vi "Parse Open Delimiter.vi"(8 "Error In":errorcluster, 11 "Parser In":refnum<class "Parser.lvclass">) -> (0 "Error Out":errorcluster, 3 "Parser Out":refnum<class "Parser.lvclass">)   [LabVIEW 2018, in "Toolkit.lvlib" / "Parser.lvclass"]
uses:
  Parser.lvclass
  Parser.lvclass/Parser.ctl
  API/Controls/States.ctl
  Tokens/Text/Text.lvclass
  D:/Users/cfield/Code/Field R&D Services/Mustache/trunk/src/Mustache/Public/Tokens/Public/Abstract/Abstract.lvclass
  Tokens/Text/API/New.vi
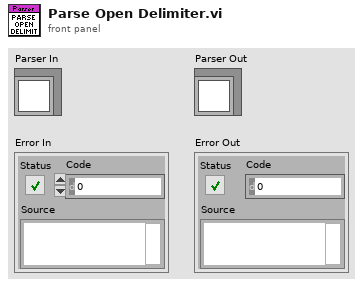
[diagram p1: front panel]
types:
  T1 = typedef "Toolkit.lvlib/Parser.lvclass/States.ctl" = enum16{"Text", "Open Delimiter", "Tag Type", "Tag Key", "Close Delimiter"}
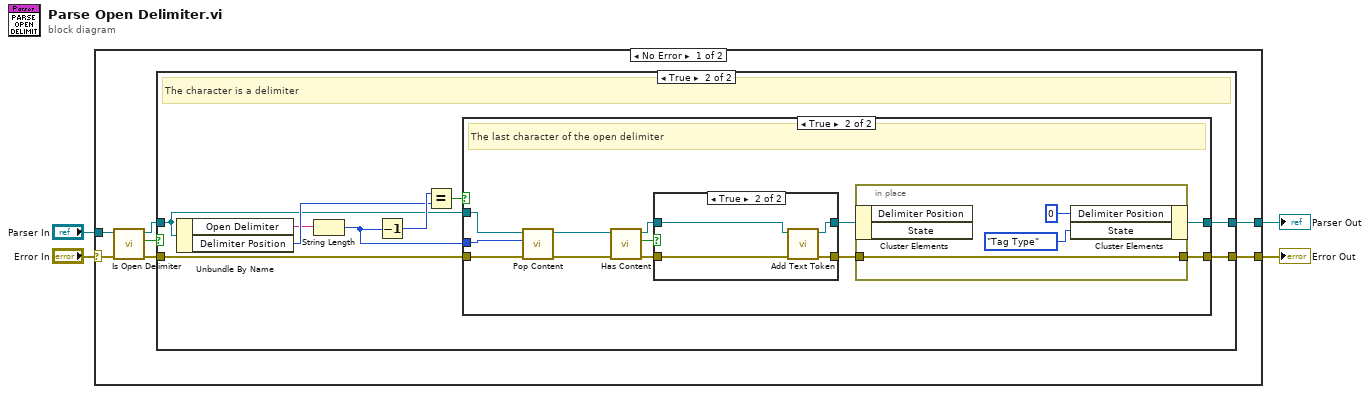
[diagram p0: block diagram]
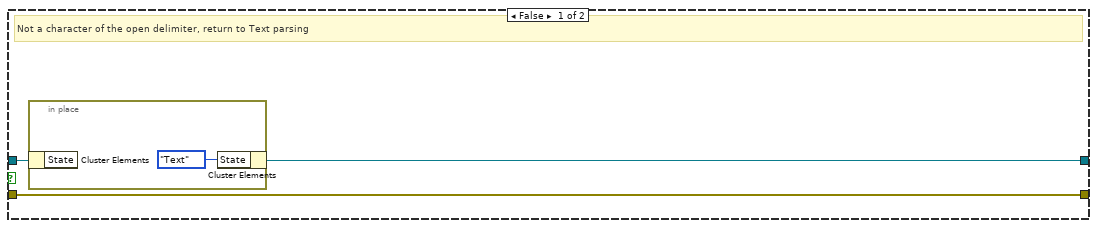
[diagram p2: hidden frame]
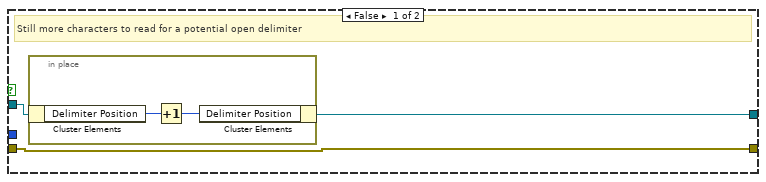
[diagram p3: hidden frame]
diagram:
  n1 = case shown="No Error" "Error In" {
    selector: "Error In" -> [w10 w51]
    tunnel: [w6 w51] -> w4
    tunnel: [w5 w52] -> w3
    tunnel: "Parser In" -> [w11 w52]
    frame No Error {
      n2 = call "Is Open Delimiter.vi"("Error In"=w10, "Parser In"=w11) -> ("Error Out"=w9:errorcluster, "Open Delimiter"=w7:bool, "Parser Out"=w8:refnum<class "Parser.lvclass">)  [unwired: 7 in]
      n3 = case shown="True" w7 {
        tunnel: w9 -> [w14 w21]
        tunnel: w8 -> [w13 w20]
        tunnel: [w14 w18] -> w6
        tunnel: [w12 w19] -> w5
        frame False {
          # "Not a character of the open delimiter, return to Text parsing"
          n4 = in-place {
            n5 = in-place-cluster #1(w13) -> ()  [unwired: 1 out]
            n6 = in-place-cluster #1("State"=States."Text") -> (w12:refnum<class "Parser.lvclass">)
          }
        }
        frame True {
          # "The character is a delimiter"
          n7 = Unbundle By Name(w20) -> ("Open Delimiter"=w17:string, "Delimiter Position"=w23:i32)
          n8 = String Length(string=w17) -> (length=w16:i32)
          n9 = Decrement(x=w16) -> (x-1=w24:i32)
          n10 = Equal?(x=w24, y=w23) -> (x = y?=w22:bool)
          n11 = case shown="True" w22 {
            tunnel: w21 -> [w25 w40]
            tunnel: w20 -> [w27 w41]
            tunnel: [w26 w34] -> w19
            tunnel: [w25 w35] -> w18
            tunnel: w16 -> [_ w39]
            frame False {
              # "Still more characters to read for a potential open delimiter"
              n12 = in-place {
                n13 = in-place-cluster #2(w27) -> ("Delimiter Position"=w29:i32)
                n14 = Increment(x=w29) -> (x+1=w28:i32)
                n15 = in-place-cluster #2("Delimiter Position"=w28) -> (w26:refnum<class "Parser.lvclass">)
              }
            }
            frame True {
              # "The last character of the open delimiter"
              n16 = call "Pop Content.vi"("Error In"=w40, "Characters Count"=w39, "Parser In"=w41) -> ("Error Out"=w32:errorcluster, "Parser Out"=w38:refnum<class "Parser.lvclass">)  [unwired: 7 in]
              n17 = call "Has Content.vi"("Error In"=w32, "Parser In"=w38) -> ("Error Out"=w31:errorcluster, "Content"=w30:bool, "Parser Out"=w33:refnum<class "Parser.lvclass">)  [unwired: 7 in]
              n18 = case shown="True" w30 {
                tunnel: [w43 w47] -> w37
                tunnel: [w42 w46] -> w36
                tunnel: w33 -> [w43 w45]
                tunnel: w31 -> [w42 w44]
                frame False {
                }
                frame True {
                  n19 = call "Add Text Token.vi"("Error In"=w44, "Parser In"=w45) -> ("Error Out"=w46:errorcluster, "Parser Out"=w47:refnum<class "Parser.lvclass">)  [unwired: 8 in]
                }
              }
              n20 = in-place {
                in-place-border: w36 -> [w50]
                in-place-border: [w50] -> w35
                n21 = in-place-cluster #3(w37) -> ()  [unwired: 2 out]
                n22 = in-place-cluster #3("Delimiter Position"=0, "State"=States."Tag Type") -> (w34:refnum<class "Parser.lvclass">)
              }
            }
          }
        }
      }
    }
    frame Error {
    }
  }
  "Error Out" <- w4
  "Parser Out" <- w3
